vi "Report App Versions.vi"(8 "error in (no error)":errorcluster, 11 "VolatusCore in":refnum<class "VolatusCore.lvclass">) -> (0 "error out":errorcluster, 3 "VolatusCore out":refnum<class "VolatusCore.lvclass">)   [LabVIEW 2020, in "Volatus.lvlib" / "VolatusCore.lvclass"]
uses:
  VolatusCore.lvclass
  VolatusCore.lvclass/VolatusCore.ctl
  VolatusConfig/VolatusConfig/VolatusConfig.lvclass
  App/App.lvclass
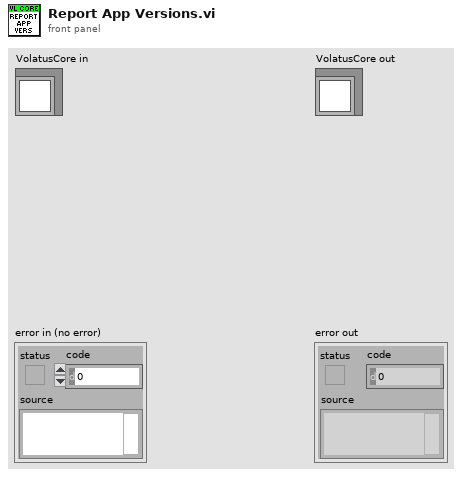
[diagram p1: front panel]
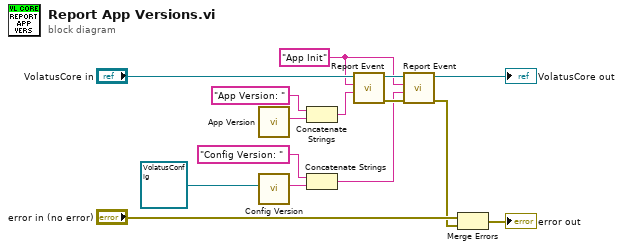
[diagram p0: block diagram]
diagram:
  w6 = "App Init" ("Context")
  n1 = call "App Version.vi"() -> ("App Version"=w11:string)  [unwired: 11 in]
  n2 = call "Config Version.vi"("VolatusConfig in"=refnum<class "VolatusConfig.lvclass"> refnum) -> ("Config Version"=w9:string)  [unwired: 8 in, 2 out]
  n3 = Concatenate Strings("App Version: ", w11) -> (w8:string)
  n4 = Concatenate Strings("Config Version: ", w9) -> (w5:string)
  n5 = call "Report Event.vi"("Message"=w8, "Context"=w6, "VolatusCore in"="VolatusCore in") -> ("error out"=w15:errorcluster, "VolatusCore out"=w7:refnum<class "VolatusCore.lvclass">)  [unwired: 7 in]
  n6 = call "Report Event.vi"("error in (no error)"=w15, "Message"=w5, "Context"=w6, "VolatusCore in"=w7) -> ("error out"=w2:errorcluster, "VolatusCore out"=→"VolatusCore out":refnum<class "VolatusCore.lvclass">)  [unwired: 6 in]
  n7 = Merge Errors("error in (no error)", w2) -> (→"error out":errorcluster)
